vi "Execute.vi"(8 "Error In":errorcluster, 10 "Command":string, 11 "Channel In":refnum<class "Channel.lvclass">) -> (0 "Error Out":errorcluster, 3 "Channel Out":refnum<class "Channel.lvclass">)   [LabVIEW 2021, in "Field_RnD_Services_LIBSSH2_Toolkit.lvlib" / "Channel.lvclass"]
doc: "Creates a single execution context for a SSH channel. To execute multiple commands, either this channel needs to be destroyed and new channel created, or a Shell channel should be used instead."
uses:
  Channel.lvclass
  Session/Session.lvclass
  Field_RnD_Services_LIBSSH2_Toolkit.lvlib
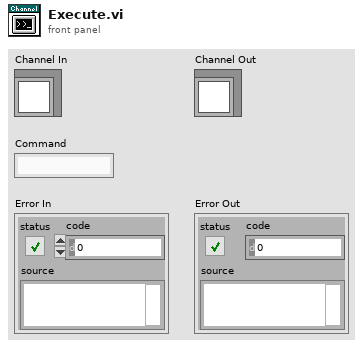
[diagram p1: front panel]
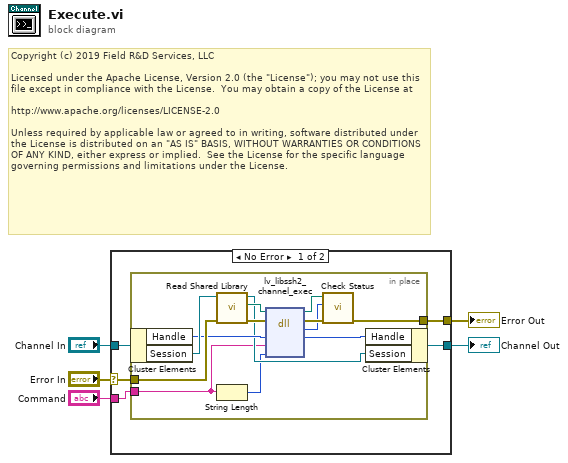
[diagram p0: block diagram]
diagram:
  # "Copyright (c) 2019 Field R&D Services, LLC\n\nLicensed under the Apache License, Version 2.0 (the \"License\"); you may not use this file except in compliance with the License.  You may obtain a copy of the License at\n\nhttp://www.apache.org/licenses/LICENSE-2.0\n\nUnless required by applicable law or agreed to in writing, software distributed under the License is distributed on an \"AS IS\" BASIS, WITHOUT WARRANTIES OR CONDITIONS OF ANY KIND, either express or implied.  See the License for the specific language governing permissions and limitations under the License."
  n1 = case shown="No Error" "Error In" {
    selector: "Error In" -> [w8 w25]
    tunnel: [w7 w25] -> w4
    tunnel: "Channel In" -> [w10 w24]
    tunnel: [w9 w24] -> w2
    tunnel: "Command" -> [w6 _]
    frame No Error {
      n2 = in-place {
        in-place-border: w8 -> [w20]
        in-place-border: [w16] -> w7
        in-place-border: w6 -> [w12]
        n3 = in-place-cluster #1(w10) -> ("Handle"=w15:u64, "Session"=w23:refnum<class "Session.lvclass">)
        n4 = call "Read Shared Library.vi"("Error In"=w20, "Session In"=w23) -> ("Erorr Out"=w21:errorcluster, "libssh2lv Shared Library"=w22:path, "Session Out"=w13:refnum<class "Session.lvclass">)  [unwired: 7 in]
        n5 = String Length(string=w12) -> (length=w11:i32)
        n6 = dll-call lib="libssh2lv.*" fn="lv_libssh2_channel_exec"(path in=w22, error in=w21, "handle"=w15, "command"=w12, "command_len"=w11) -> (path out=w18:path, error out=w19:errorcluster, "status"=w17:i32, "handle"=w14:u64)  [unwired: 3 in]
        n7 = call "Check Status.vi"("Error In"=w19, "Status"=w17, "libssh2lv Shared Library In"=w18) -> ("Error Out"=w16:errorcluster)  [unwired: 7 in, 1 out]
        n8 = in-place-cluster #1("Handle"=w14, "Session"=w13) -> (w9:refnum<class "Channel.lvclass">)
      }
    }
    frame Error {
    }
  }
  "Error Out" <- w4
  "Channel Out" <- w2
